vi "punto #4.vi"() -> ()   [LabVIEW 2017]
panel:
  in  "star":bool
  out "lleg. iz":bool
  out "lleg. der":bool
  in  "velocidad (m/300ms)":dbl(knob) scale=0.0..10.0
  in  "direccion":bool
  out "banda":dbl(slide) scale=0.0..1200.0
  # "derecha"
  # "izquierda"
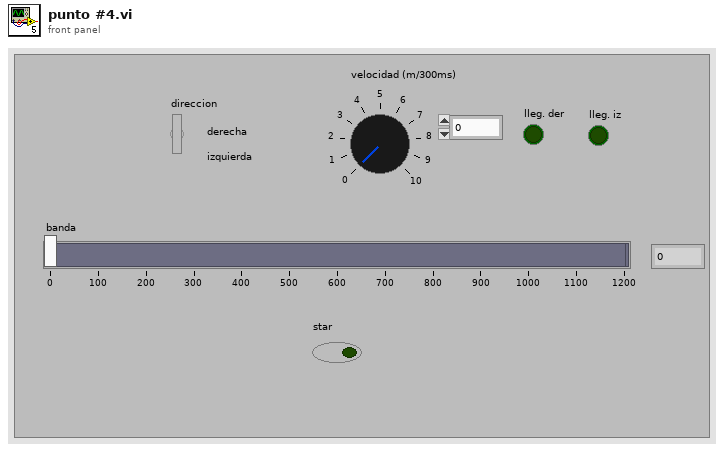
[diagram p1: front panel]
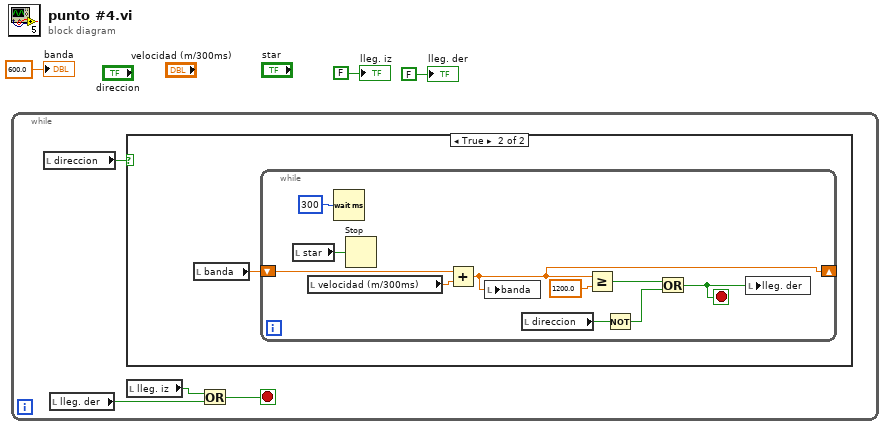
[diagram p0: block diagram]
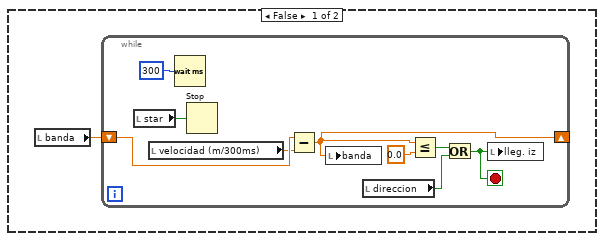
[diagram p2: hidden frame]
diagram:
  n1 = while {
    stop <- w6 stop-if-true
    n2 = local read "direccion"() -> (w7:bool)
    n3 = local read "lleg. der"() -> (w4:bool)
    n4 = case shown="True" w7 {
      frame False {
        n5 = local read "banda"() -> (w8:dbl)
        n6 = while {
          shift-right: [w14] -> _
          shift-left: w8 -> [w17]
          stop <- w11 stop-if-true
          n7 = local read "star"() -> (w9:bool)
          n8 = local read "velocidad (m/300ms)"() -> (w16:dbl)
          n9 = Wait (ms)(milliseconds to wait=u32 300) -> ()  [unwired: 1 out]
          n10 = Stop(stop? (T)=w9) -> ()
          n11 = Subtract(x=w17, y=w16) -> (x-y=w14:dbl)
          n12 = local write "banda"(w14) -> ()
          n13 = local read "direccion"() -> (w10:bool)
          n14 = Less Or Equal?(x=w14, y=0.0) -> (x <= y?=w13:bool)
          n15 = Or(x=w13, y=w10) -> (x .or. y?=w11:bool)
          n16 = local write "lleg. iz"(w11) -> ()
        }
      }
      frame True {
        n17 = local read "banda"() -> (w18:dbl)
        n18 = while {
          shift-right: [w26] -> _
          shift-left: w18 -> [w28]
          stop <- w21 stop-if-true
          n19 = local read "star"() -> (w19:bool)
          n20 = local read "velocidad (m/300ms)"() -> (w27:dbl)
          n21 = Wait (ms)(milliseconds to wait=u32 300) -> ()  [unwired: 1 out]
          n22 = Stop(stop? (T)=w19) -> ()
          n23 = Add(x=w28, y=w27) -> (x+y=w26:dbl)
          n24 = local write "banda"(w26) -> ()
          n25 = local read "direccion"() -> (w23:bool)
          n26 = Greater Or Equal?(x=w26, y=1200.0) -> (x >= y?=w24:bool)
          n27 = Not(x=w23) -> (.not. x?=w20:bool)
          n28 = Or(x=w24, y=w20) -> (x .or. y?=w21:bool)
          n29 = local write "lleg. der"(w21) -> ()
        }
      }
    }
    n30 = local read "lleg. iz"() -> (w5:bool)
    n31 = Or(x=w5, y=w4) -> (x .or. y?=w6:bool)
  }
  "banda" <- 600.0 ("banda")
  "lleg. iz" <- FALSE ("lleg. iz")
  "lleg. der" <- FALSE ("lleg. der")
